vi "AutomatedBeamGage_Instance.vi"() -> ()   [LabVIEW 2018]
uses:
  C:/Program Files/Spiricon/BeamSquared/M2.Automation.dll
  M2.Automation.dll
panel:
  out "AutomatedBeamSquared":refnum<k24>
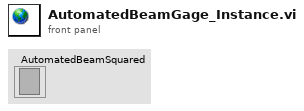
[diagram p1: front panel]
diagram:
